vi "add_vectors.vi"(0 "vector_qdrant in":refnum<class "vector_qdrant.lvclass">, 5 "colection_name":string, 7 "vectors":T1[](array[typedef]), 11 "error in (no error)":errorcluster) -> (4 "vector_qdrant out":refnum<class "vector_qdrant.lvclass">, 15 "error out":errorcluster)   [LabVIEW 2020, in "vector_qdrant.lvclass"]
uses:
  vector_qdrant.lvclass
  abstract_vector_base/vector.ctl
  vector_qdrant.lvclass/vector_qdrant.ctl
  <vilib>/httpClient/PUTBuffer.vi
  <vilib>/httpClient/LabVIEWHTTPClient.lvlib
  abstract_vector_base/abstract_vector_base.lvclass
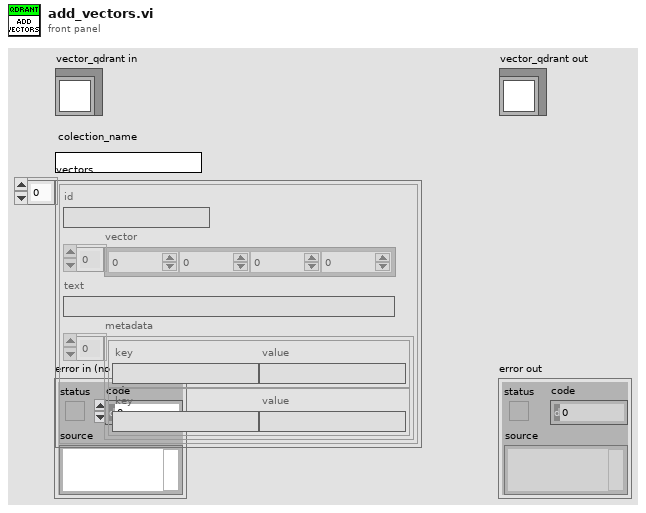
[diagram p1: front panel]
types:
  T1 = typedef "abstract_vector_base.lvclass/vector.ctl" = cluster{"id":string, "vector":dbl[], "text":string, "metadata":cluster{"key":string, "value":string}[]}
  T2 = cluster{"batch":cluster{"ids":string[], "vectors":dbl[][], "payloads":cluster{"text":string}[]}}
  T3 = cluster{"points":cluster{"id":string, "vector":dbl[], "payload":cluster{"text":string, "metadata":cluster{"key":string, "value":string}[]}}[]}
  T4 = typedef "LabVIEWHTTPClient.lvlib/ClientHandle.ctl" = refnum<k1>
  T5 = cluster{"id":string, "vector":dbl[], "payload":cluster{"text":string, "metadata":cluster{"key":string, "value":string}[]}}
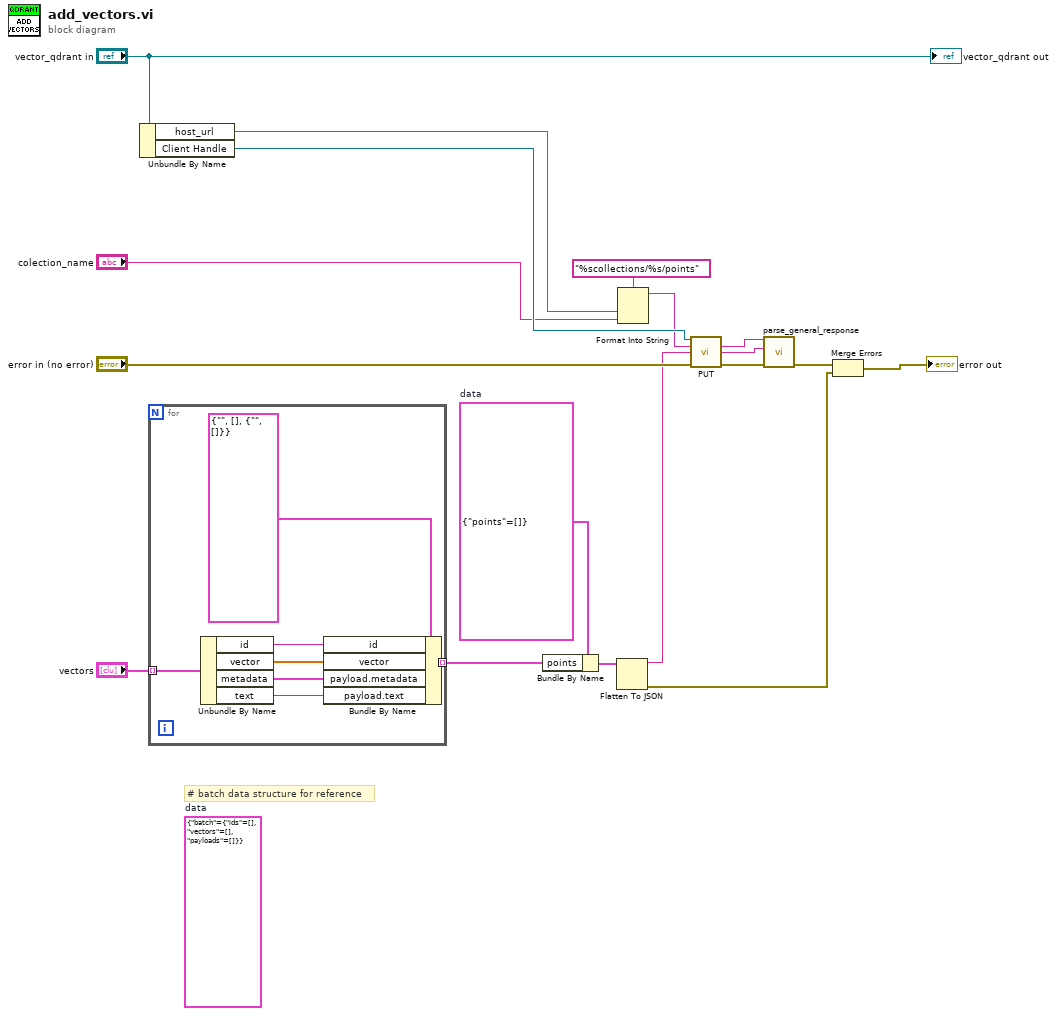
[diagram p0: block diagram]
diagram:
  (unwired) T2 {"batch"={"ids"=[], "vectors"=[], "payloads"=[]}}  # data
  w3 = T3 {"points"=[]}  # data
  # "# batch data structure for reference"
  n1 = Unbundle By Name("vector_qdrant in") -> ("host_url"=w17:string, "Client Handle"=w15:T4)
  n2 = for {
    tunnel: "vectors" -> [w25] mode=indexing
    tunnel: [w21] -> w1 mode=indexing
    n3 = Unbundle By Name(w25) -> ("id"=w23:string, "vector"=w22:dbl[], "metadata"=w20:cluster{"key":string, "value":string}[], "text"=w19:string)
    n4 = Bundle By Name(cluster=T5 {"id"="", "vector"=[], "payload"={"text"="", "metadata"=[]}} ("point"), "id"=w23, "vector"=w22, "payload.metadata"=w20, "payload.text"=w19) -> (w21:T5)
  }
  n5 = Bundle By Name(cluster=w3, "points"=w1) -> (w2:T3)
  n6 = Flatten To JSON(anything=w2) -> (JSON string=w6:string, 11:w4:errorcluster)  [unwired: 2 in]
  n7 = Format Into String(format string="%scollections/%s/points", w17, "colection_name") -> (resulting string=w14:string)  [unwired: 2 in, 1 out]
  n8 = call-poly <vilib>:"PUT.vi"("client handle"=w15, "url"=w14, "buffer"=w6, "error in (no error)"="error in (no error)") -> ("headers"=w11:string, "body"=w10:string, "error out"=w12:errorcluster)  [unwired: 8 in, 1 out]
  n9 = call "parse_general_response.vi"("error in (no error)"=w12, "body"=w10, "headers"=w11) -> ("error out"=w9:errorcluster)  [unwired: 8 in]
  n10 = Merge Errors(w9, w4) -> (→"error out":errorcluster)
  "vector_qdrant out" <- "vector_qdrant in"
